vi "Untitled 1.vi"   [LabVIEW 2019]
uses:
  <vilib>/imath/engines/lvmath2/RunTimeEngine/NodeEndStatement/NIMS_NodeEndStatement_Output.vi
  <vilib>/imath/engines/lvmath2/RunTimeEngine/ErrorHandling/NIMS_Finalize Error.vi
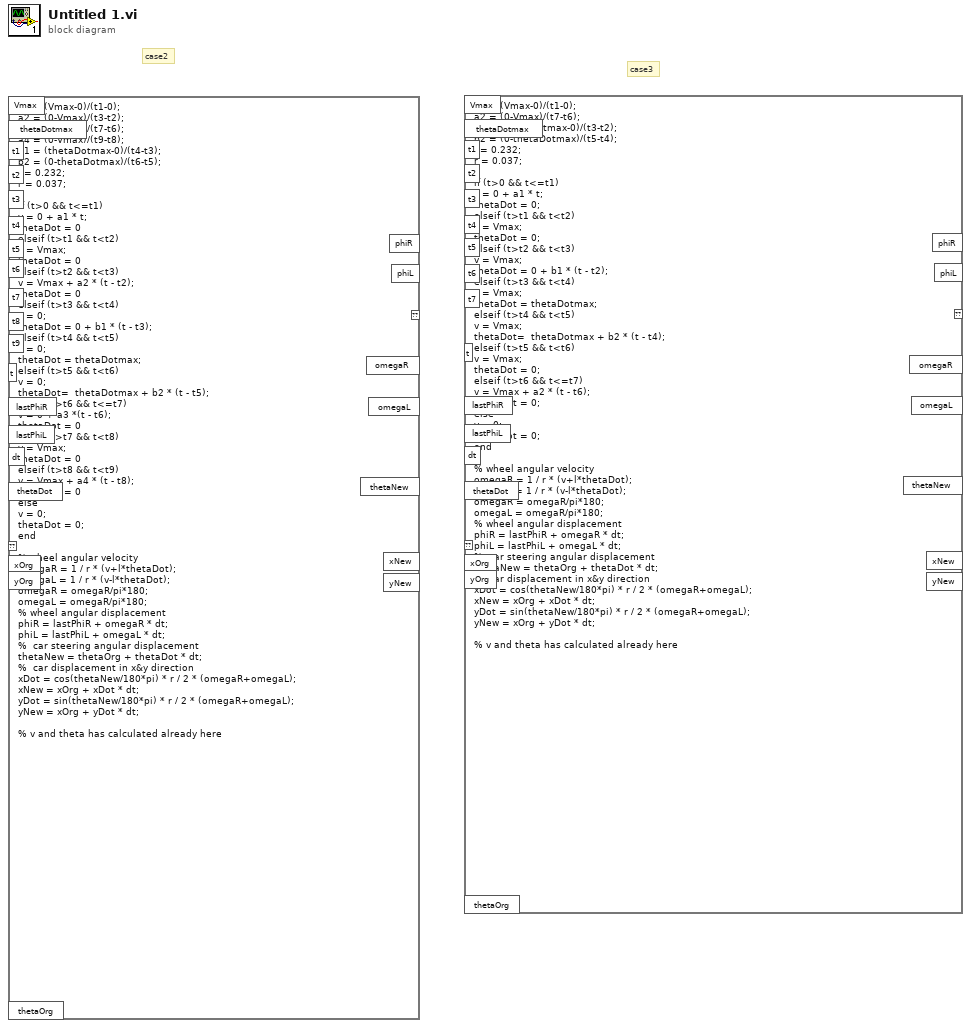
[diagram p0: block diagram]
diagram:
  # "case3"
  # "case2"
  n1 = mathscript code="a1 = (Vmax-0)/(t1-0);\na2 = (0-Vmax)/(t3-t2);\na3 = (Vmax-0)/(t7-t6); \na4 = (0-Vmax)/(t9-t8);\nb1 = (thetaDotmax-0)/(t4-t3);\nb2 = (0-thetaDotmax)/(t6-t5); \nl = 0.232;\nr = 0.037;\n\nif (t>0 && t<=t1)\nv = 0 + a1 * t;\nthetaDot = 0\nelseif (t>t1 && t<t2)\nv = Vmax;\nthetaDot = 0\nelseif (t>t2 && t<t3)\nv = Vmax + a2 * (t - t2);\nthetaDot = 0\nelseif (t>t3 && t<t4)\nv = 0;\nthetaDot = 0 + b1 * (t - t3);\nelseif (t>t4 && t<t5)\nv = 0;\nthetaDot = thetaDotmax;\nelseif (t>t5 && t<t6)\nv = 0;\nthetaDot=  thetaDotmax + b2 * (t - t5);\nelseif (t>t6 && t<=t7)\nv = 0 + a3 *(t - t6);\nthetaDot = 0\nelseif (t>t7 && t<t8)\nv = Vmax;\nthetaDot = 0\nelseif (t>t8 && t<t9)\nv = Vmax + a4 * (t - t8);\nthetaDot = 0\nelse\nv = 0;\nthetaDot = 0;\nend\n\n% wheel angular velocity \nomegaR = 1 / r * (v+l*thetaDot);\nomegaL = 1 / r * (v-l*thetaDot);\nomegaR = omegaR/pi*180;\nomegaL = omegaR/pi*180;\n% wheel angular displacement\nphiR = lastPhiR + omegaR * dt;\nphiL = lastPhiL + omegaL * dt;\n%  car steering angular displacement\nthetaNew = thetaOrg + thetaDot * dt;\n%  car displacement in x&y direction\nxDot = cos(thetaNew/180*pi) * r / 2 * (omegaR+omegaL);\nxNew = xOrg + xDot * dt;\nyDot = sin(thetaNew/180*pi) * r / 2 * (omegaR+omegaL);\nyNew = xOrg + yDot * dt;\n\n% v and theta has calculated already here"() -> ()  [unwired: 20 in, 8 out]
  n2 = mathscript code="a1 = (Vmax-0)/(t1-0);\na2 = (0-Vmax)/(t7-t6);\nb1 = (thetaDotmax-0)/(t3-t2);\nb2 = (0-thetaDotmax)/(t5-t4); \nl = 0.232;\nr = 0.037;\n\nif (t>0 && t<=t1)\nv = 0 + a1 * t;\nthetaDot = 0;\nelseif (t>t1 && t<t2)\nv = Vmax;\nthetaDot = 0;\nelseif (t>t2 && t<t3)\nv = Vmax;\nthetaDot = 0 + b1 * (t - t2);\nelseif (t>t3 && t<t4)\nv = Vmax;\nthetaDot = thetaDotmax;\nelseif (t>t4 && t<t5)\nv = Vmax;\nthetaDot=  thetaDotmax + b2 * (t - t4);\nelseif (t>t5 && t<t6)\nv = Vmax;\nthetaDot = 0;\nelseif (t>t6 && t<=t7)\nv = Vmax + a2 * (t - t6);\nthetaDot = 0;\nelse\nv = 0;\nthetaDot = 0;\nend\n\n% wheel angular velocity \nomegaR = 1 / r * (v+l*thetaDot);\nomegaL = 1 / r * (v-l*thetaDot);\nomegaR = omegaR/pi*180;\nomegaL = omegaR/pi*180;\n% wheel angular displacement\nphiR = lastPhiR + omegaR * dt;\nphiL = lastPhiL + omegaL * dt;\n%  car steering angular displacement\nthetaNew = thetaOrg + thetaDot * dt;\n%  car displacement in x&y direction\nxDot = cos(thetaNew/180*pi) * r / 2 * (omegaR+omegaL);\nxNew = xOrg + xDot * dt;\nyDot = sin(thetaNew/180*pi) * r / 2 * (omegaR+omegaL);\nyNew = xOrg + yDot * dt;\n\n% v and theta has calculated already here"() -> ()  [unwired: 18 in, 8 out]
